vi "PH_PPMA_PowerUnit.src Ross.vi"(0 "i ref in":refnum<vi>, 5 "error in (no error)":errorcluster) -> (14 "i ref out":refnum<vi>, 19 "error out":errorcluster)   [LabVIEW 2014, in "PH_PPMA_PowerUnit.lvlib"]
doc: "This is the action VI of the _StateRoss event case. It checks the Device state. Depending on this the following is done:\n\n1 (RR closed): if SM State = \"Open Ross Relais\" and Ignitron.State Device = on and State Rel Rods = on (up) and State PSU = off, a state change request is send to SM to get \"Switch GD Channel on\"\n2 (RR open): if SM State = \"Close Ross Relais\" and Ignitron.State Device = on and State Rel Rods = on (up) and State PSU = off, a state change request is send to SM to get \"Switch PSU on\"\n\nIt finally calls \"State PU\"."
uses:
  PH_PPMA_PowerUnit.lvlib
  PH_StatusHandler/PH_StatusHandler.Status.ctl
  PH_PowerUnit_BaseClass/PH_PowerUnit_BaseClass.SM States.ctl
  PH_PowerUnit_BaseClass/PH_PowerUnit_BaseClass.lvlib
  PH_StatusHandler/PH_StatusHandler.lvlib
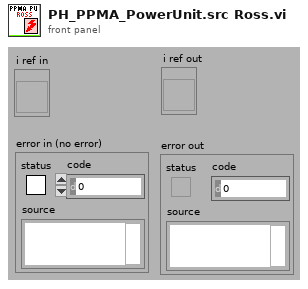
[diagram p1: front panel]
types:
  T1 = typedef "PH_StatusHandler.lvlib/PH_StatusHandler.Status.ctl" = i16
  T2 = typedef "PH_PPMA_PowerUnit.lvlib/PH_PPMA_PowerUnit.i attribute.ctl" = cluster{"GUI Refs":cluster{"Rods":refnum<vi>, "Ignitron":refnum<vi>, "Rossrelais":refnum<vi>, "Set Voltage":refnum<vi>, "PSU":refnum<vi>, "EOC":refnum<vi>, "Trigger":refnum<vi>}, "Rods":T3, "PSU":T4, "Ross Relais":T5, "Ignitron":T6, "Trigger":cluster{"State Device":T1, "linked?":bool}, "Timing Settings":cluster{"Prdc Fast?":bool, "Default Value Periodic Interval":i32, "Mercury on since":dbl, "Warm up Time Mercury [s]":dbl}, "Set Voltage [V]":dbl}
  T3 = typedef "PH_PPMA_PowerUnit.lvlib/PH_PPMA_PowerUnit.Rods Attributes.ctl" = cluster{"Instancename":string, "Device Status":T1, "linked?":bool}
  T4 = typedef "PH_PP_Common.lvlib/PH_PP_Common.PSU Attributes.ctl" = cluster{"lower limit [V]":dbl, "upper limit [V]":dbl, "Voltage set":bool, "State Device":T1, "linked?":bool}
  T5 = typedef "PH_PP_Common.lvlib/PH_PP_Common.Ross Relais Attributes.ctl" = cluster{"State Device":T1, "linked?":bool}
  T6 = typedef "PH_PP_Common.lvlib/PH_PP_Common.Ignitron Attributes.ctl" = cluster{"State Device":T1, "linked?":bool}
  T7 = typedef "PH_PowerUnit_BaseClass.lvlib/PH_PowerUnit_BaseClass.SM States.ctl" = enum16{".", "Stand by", "Switch PU on", "Configure", "Set Default Voltage", "Set STANDBY", "Set READY", "Wait for Shot Cmd", "Open Dump Rods", "Open Ross Relais", "Close Ross Relais", "Switch PSU on", "Switch PSU off", "Charge", "Switch GD Channel on", "Close Dump Rods", "Rods-TO", "RR-TO", "PSU-TO", "Trigger-TO"}
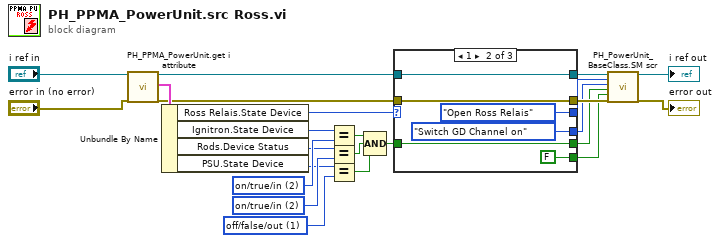
[diagram p0: block diagram]
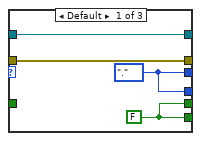
[diagram p2: hidden frame]
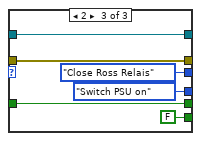
[diagram p3: hidden frame]
diagram:
  w16 = T1 1 items=["no info", "off/false/out", "on/true/in", "Failure", "Alarm", "Status 1", "Status 2", "Status 3"] ("PSU.State PSU")
  w17 = T1 2 items=["no info", "off/false/out", "on/true/in", "Failure", "Alarm", "Status 1", "Status 2", "Status 3"] ("Rods.State Rel Rods")
  w18 = T1 2 items=["no info", "off/false/out", "on/true/in", "Failure", "Alarm", "Status 1", "Status 2", "Status 3"] ("Ignitron.State Device")
  n1 = call "PH_PPMA_PowerUnit.get i attribute.vi"("i ref in"="i ref in", "error in (no error)"="error in (no error)") -> ("i ref out"=w21:refnum<vi>, "i attribute"=w24:T2, "error out"=w20:errorcluster)  [unwired: 15 in]
  n2 = Unbundle By Name(w24) -> ("Ross Relais.State Device"=w19:T1, "Ignitron.State Device"=w15:T1, "Rods.Device Status"=w14:T1, "PSU.State Device"=w13:T1)
  n3 = Equal?(x=w15, y=w18) -> (x = y?=w12:bool)
  n4 = Equal?(x=w14, y=w17) -> (x = y?=w11:bool)
  n5 = Equal?(x=w13, y=w16) -> (x = y?=w10:bool)
  n6 = Compound Arithmetic op=AND(w12, w11, w10) -> (w9:bool)
  n7 = case shown="1" w19 {
    tunnel: w21 -> [w28 w30 w36]
    tunnel: w20 -> [w27 w29 w35]
    tunnel: [w27 w29 w35] -> w8
    tunnel: [w28 w30 w36] -> w6
    tunnel: w9 -> [_ w34 w40]
    tunnel: [w25 w34 w40] -> w4
    tunnel: [w26 PH_PowerUnit_BaseClass.SM_States."Open Ross Relais" ("Current SM State (condition)") PH_PowerUnit_BaseClass.SM_States."Close Ross Relais" ("Current SM State (condition)")] -> w3
    tunnel: [w26 PH_PowerUnit_BaseClass.SM_States."Switch GD Channel on" ("Current SM State (condition)") PH_PowerUnit_BaseClass.SM_States."Switch PSU on" ("Current SM State (condition)")] -> w2
    tunnel: [w25 FALSE ("PU in use is condition? (true)") FALSE ("PU in use is condition? (true)")] -> w1
    frame Default {
      w25 = FALSE ("PU in use is condition? (true)")
      w26 = PH_PowerUnit_BaseClass.SM_States."." ("Current SM State (condition)")
    }
    frame 1 {
    }
    frame 2 {
    }
  }
  n8 = call "PH_PowerUnit_BaseClass.SM scr.vi"("VI in"=w6, "Current SM State (condition)"=w3, "Wanted SM State"=w2, "Further change condition"=w4, "PU in use is condition? (true)"=w1, "error in (no error)"=w8) -> ("VI out"=→"i ref out":refnum<vi>, "error out"=→"error out":errorcluster)  [unwired: 12 in]
